vi "Launch.vi"   [LabVIEW 2018]
uses:
  Calling Actor/Calling Actor.lvclass
  C:/Program Files (x86)/National Instruments/LabVIEW 2018/vi.lib/ActorFramework/Actor/Actor.lvclass
  <vilib>/ActorFramework/Actor/Actor.lvclass
types:
  T1 = enum32{"Invalid", "Standard", "Closed", "Hidden", "Minimized", "Maximized"}
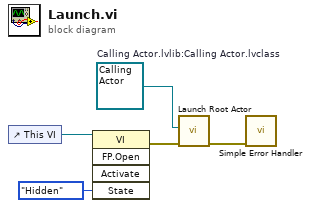
[diagram p0: block diagram]
diagram:
  w5 = refnum<class "Calling Actor.lvclass"> refnum  # Calling Actor.lvlib:Calling Actor.lvclass
  n1 = control-ref of="This VI"() -> (w1:refnum<vi>)
  n2 = invoke class="VI" method="FP.Open"(reference=w1, "State"=T1."Hidden") -> (error out=w2:errorcluster)  [unwired: 3 in, 4 out]
  n3 = call <vilib>:"Launch Root Actor.vi"("error in (no error)"=w2, "Actor"=w5) -> ("error out"=w4:errorcluster)  [unwired: 8 in, 1 out]
  n4 = call <vilib>:"Simple Error Handler.vi"("error in (no error)"=w4) -> ()  [unwired: 4 in, 5 out]
